vi "If GObject Reference Equal.vi"(8 "error in (no error)":errorcluster, 10 "GObjects":refnum<vi>[](array[refnum]), 11 "GObject in":refnum<class "Object.lvclass">) -> (0 "error out":errorcluster, 2 "Index Found":i32, 3 "GObject out":refnum<class "Object.lvclass">)   [LabVIEW 2015, in "Front Panel Publisher.lvlib" / "Object.lvclass"]
uses:
  Object.lvclass
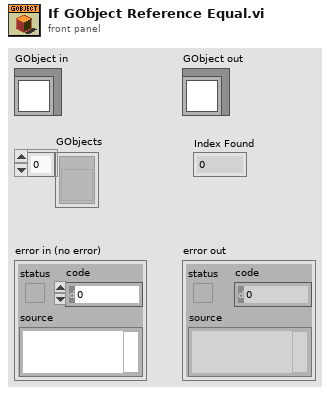
[diagram p1: front panel]
types:
  T1 = typedef "Front Panel Publisher.lvlib/Object.lvclass/Attributes.ctl" = cluster{"UID":i32, "Type":string, "Coordinates":T2, "Reference":refnum<vi>}
  T2 = typedef "Front Panel Publisher.lvlib/Object.lvclass/Coordinates.ctl" = cluster{"Left":i32, "Top":i32, "Height":u32, "Width":u32}
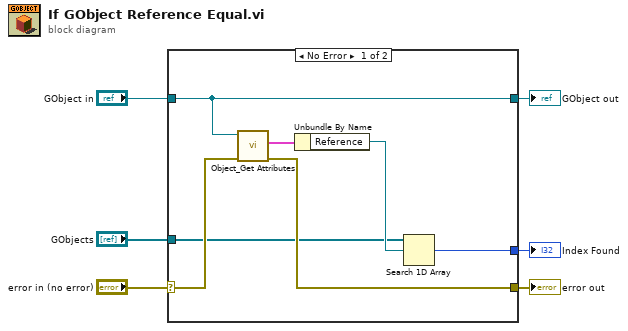
[diagram p0: block diagram]
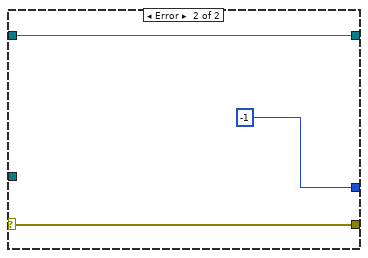
[diagram p2: hidden frame]
diagram:
  n1 = case shown="No Error" "error in (no error)" {
    selector: "error in (no error)" -> [w10 w16]
    tunnel: [w9 w16] -> w5
    tunnel: [w13 w15] -> w3
    tunnel: "GObject in" -> [w13 w15]
    tunnel: "GObjects" -> [w8 _]
    tunnel: [w7 -1 ("index of element")] -> w1
    frame No Error {
      n2 = call "Object_Get Attributes.vi"("error in (no error)"=w10, "Object In"=w13) -> ("error out"=w9:errorcluster, "Data"=w12:T1)  [unwired: 6 in, 2 out]
      n3 = Unbundle By Name(w12) -> ("Reference"=w11:refnum<vi>)
      n4 = Search 1D Array(1D array=w8, element=w11) -> (index of element=w7:i32)  [unwired: 1 in]
    }
    frame Error {
    }
  }
  "error out" <- w5
  "GObject out" <- w3
  "Index Found" <- w1
